vi "Dynamic Offset.vi"(8 "error in (no error)":errorcluster, 9 "Top Offset (%)":dbl, 10 "Left Offset (%)":dbl, 11 "Position":T1) -> (0 "error out":errorcluster, 3 "Offset Positon":T1)   [LabVIEW 2014]
uses:
  <vilib>/Utility/miscctls.llb/LVPositionTypeDef.ctl
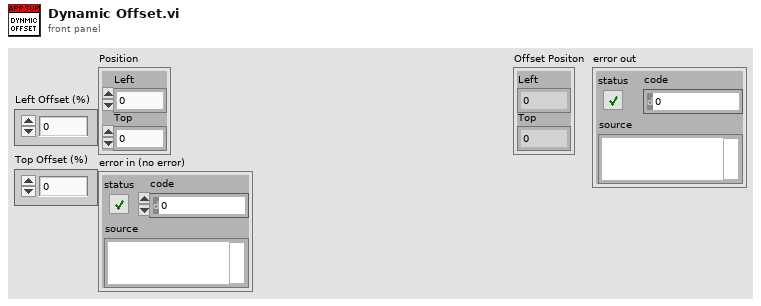
[diagram p1: front panel]
types:
  T1 = typedef "LVPositionTypeDef.ctl" = cluster{"Left":i32, "Top":i32}
  T2 = typedef "LVRectTypeDef.ctl" = cluster{"Left":i16, "Top":i16, "Right":i16, "Bottom":i16}
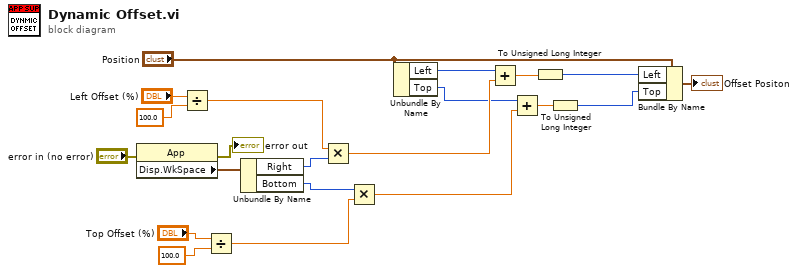
[diagram p0: block diagram]
diagram:
  n1 = property class="App"(error in="error in (no error)") -> (error out=→"error out":errorcluster, "Disp.WkSpace"=w20:T2)  [unwired: 1 in, 1 out]
  n2 = Divide(x="Left Offset (%)", y=100.0) -> (x/y=w14:dbl)
  n3 = Divide(x="Top Offset (%)", y=100.0) -> (x/y=w12:dbl)
  n4 = Unbundle By Name(w20) -> ("Right"=w15:i16, "Bottom"=w13:i16)
  n5 = Multiply(x=w14, y=w15) -> (x*y=w10:dbl)
  n6 = Multiply(x=w13, y=w12) -> (x*y=w8:dbl)
  n7 = Unbundle By Name("Position") -> ("Left"=w11:i32, "Top"=w9:i32)
  n8 = Add(x=w11, y=w10) -> (x+y=w7:dbl)
  n9 = Add(x=w9, y=w8) -> (x+y=w6:dbl)
  n10 = To Unsigned Long Integer(number=w7) -> (unsigned 32bit integer=w4:u32)
  n11 = To Unsigned Long Integer(number=w6) -> (unsigned 32bit integer=w3:u32)
  n12 = Bundle By Name(cluster="Position", "Left"=w4, "Top"=w3) -> (→"Offset Positon":T1)
